vi "fileRenameAddDate.vi"(9 "name or relative path":string, 11 "base path":path) -> ()   [LabVIEW 2012]
panel:
  out "error out":errorcluster
  out "Destination":path
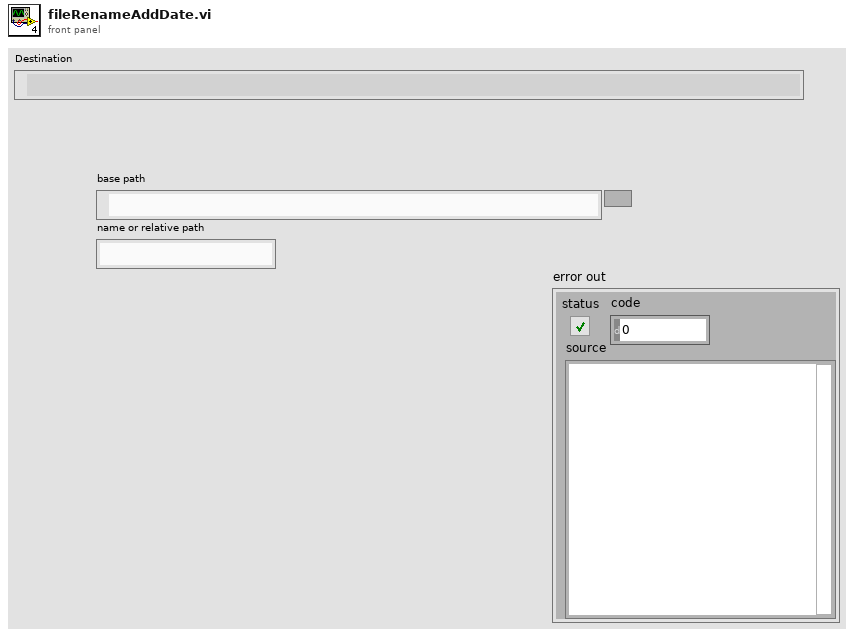
[diagram p1: front panel]
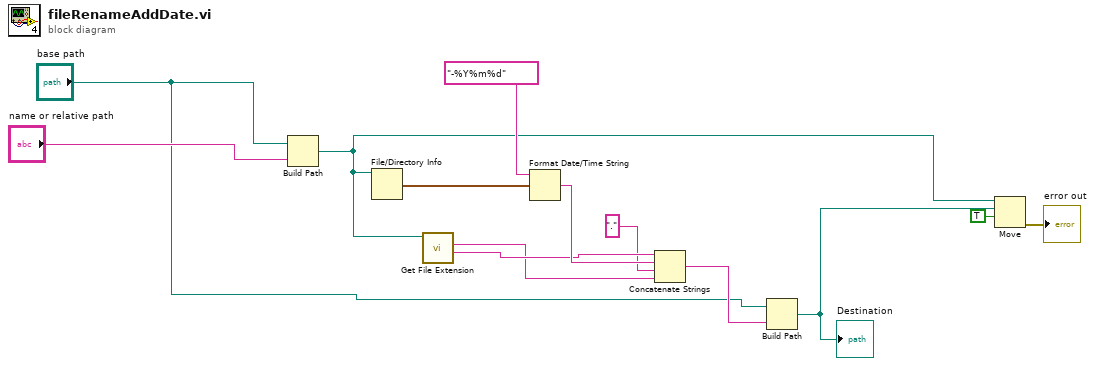
[diagram p0: block diagram]
diagram:
  n1 = Build Path(base path="base path", name or relative path="name or relative path") -> (appended path=w6:path)
  n2 = File/Directory Info(path=w6) -> (last mod=w12:timestamp)  [unwired: 1 in, 6 out]
  n3 = call <vilib>:"Get File Extension.vi"("file"=w6) -> ("filename without extension"=w5:string, "lowercase file extension"=w3:string)  [unwired: 7 in, 2 out]
  n4 = Format Date/Time String(time format string (%c)="-%Y%m%d", seconds (now)=w12) -> (date/time string=w10:string)  [unwired: 1 in]
  n5 = Concatenate Strings(w5, w10, "." ("string"), w3) -> (w2:string)
  n6 = Build Path(base path="base path", name or relative path=w2) -> (appended path=w9:path)
  "Destination" <- w9
  n7 = Move(source path=w6, 9:TRUE ("overwrite (F)"), 10:w9) -> (error out=→"error out":errorcluster)  [unwired: 2 in, 2 out]
